vi "Mouse In.vi"(8 "error in (no error)":errorcluster, 10 "MousePoint":cluster{"x":i16, "y":i16}, 11 "Line in":refnum<class "Line.lvclass">) -> (0 "error out":errorcluster, 2 "In?":bool, 3 "Line out":refnum<class "Line.lvclass">)   [LabVIEW 2015, in "Line.lvclass"]
uses:
  Line.lvclass
  Graphic/Graphic.lvclass/Graphic.ctl
  Graphic/Graphic.lvclass
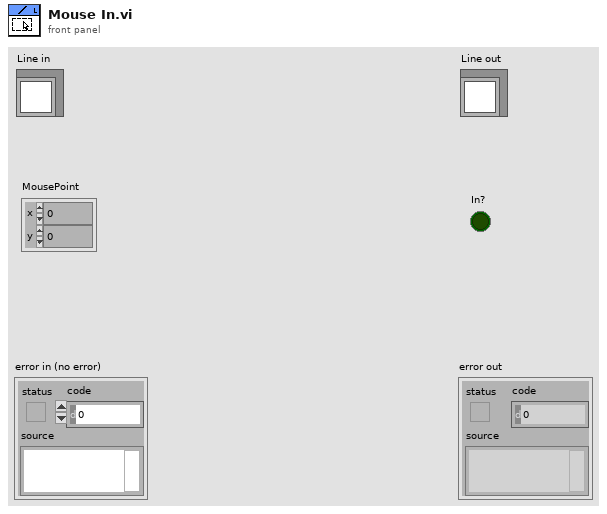
[diagram p1: front panel]
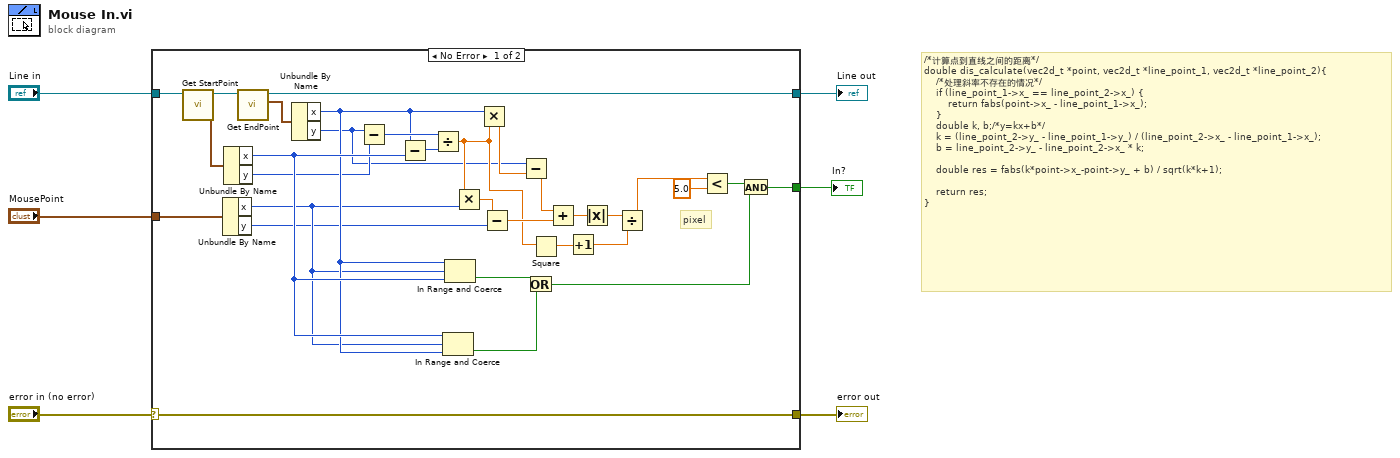
[diagram p0: block diagram]
diagram:
  # "/*计算点到直线之间的距离*/\ndouble dis_calculate(vec2d_t *point, vec2d_t *line_point_1, vec2d_t *line_point_2){\n    /*处理斜率不存在的情况*/\n    if (line_point_1->x_ == line_point_2->x_) {\n        return fabs(point->x_ - line_point_1->x_);\n    }\n    double k, b;/*y=kx+b*/\n    k = (line_point_2->y_ - line_point_1->y_) / (line_point_2->x_ - line_point_1->x_);\n    b = line_point_2->y_ - line_point_2->x_ * k;\n    \n    double res = fabs(k*point->x_-point->y_ + b) / sqrt(k*k+1);\n \n    return res;\n}"
  n1 = case shown="No Error" "error in (no error)" {
    selector: "error in (no error)" -> [w37 w39]
    tunnel: "Line in" -> [w36 w38]
    tunnel: [w34 w38] -> w4
    tunnel: "MousePoint" -> [w33 _]
    tunnel: [w37 w39] -> w2
    tunnel: [w10 _] -> w1
    frame No Error {
      # "pixel"
      n2 = call "Get StartPoint.vi"("Graphic in"=w36) -> ("StartPoint"=w32:cluster{"x":i16, "y":i16}, "Graphic out"=w35:refnum<class "Line.lvclass">)  [unwired: 8 in, 1 out]
      n3 = Unbundle By Name(w33) -> ("x"=w15:i16, "y"=w12:i16)
      n4 = Unbundle By Name(w32) -> ("x"=w17:i16, "y"=w14:i16)
      n5 = call "Get EndPoint.vi"("Graphic in"=w35) -> ("EndPoint"=w31:cluster{"x":i16, "y":i16}, "Graphic out"=w34:refnum<class "Line.lvclass">)  [unwired: 8 in, 1 out]
      n6 = Unbundle By Name(w31) -> ("x"=w16:i16, "y"=w13:i16)
      n7 = Subtract(x=w13, y=w14) -> (x-y=w29:i16)
      n8 = Subtract(x=w16, y=w17) -> (x-y=w28:i16)
      n9 = Divide(x=w29, y=w28) -> (x/y=w21:dbl)
      n10 = In Range and Coerce(upper limit=w17, x=w15, lower limit=w16) -> (In Range?=w8:bool)  [unwired: 1 out]
      n11 = In Range and Coerce(upper limit=w16, x=w15, lower limit=w17) -> (In Range?=w9:bool)  [unwired: 1 out]
      n12 = Multiply(x=w21, y=w15) -> (x*y=w27:dbl)
      n13 = Multiply(x=w16, y=w21) -> (x*y=w26:dbl)
      n14 = Subtract(x=w27, y=w12) -> (x-y=w25:dbl)
      n15 = Subtract(x=w13, y=w26) -> (x-y=w24:dbl)
      n16 = Or(x=w9, y=w8) -> (x .or. y?=w7:bool)
      n17 = Square(x=w21) -> (x^2=w20:dbl)
      n18 = Add(x=w24, y=w25) -> (x+y=w23:dbl)
      n19 = Increment(x=w20) -> (x+1=w19:dbl)
      n20 = Absolute Value(x=w23) -> (abs(x)=w22:dbl)
      n21 = Divide(x=w22, y=w19) -> (x/y=w18:dbl)
      n22 = Less?(x=w18, y=5.0) -> (x < y?=w11:bool)
      n23 = And(x=w11, y=w7) -> (x .and. y?=w10:bool)
    }
    frame Error {
    }
  }
  "error out" <- w2
  "Line out" <- w4
  "In?" <- w1
